vi "QPSK.vi"() -> ()   [LabVIEW 2018]
uses:
  <vilib>/addons/Modulation/Digital/General/MT Generate Bits (Galois, PN Order).vi
  <vilib>/addons/Modulation/Digital/Support/Common/Validators/mod_Generate Bits Validate.vi
  <vilib>/addons/Modulation/Analog/support/mod_Set Error Source.vi
  <vilib>/addons/Modulation/Digital/General/subVIs/mod_Generate Bits PN Sequence.vi
  <vilib>/addons/Modulation/niDMT.lvlib
panel:
  out "complex symbols":cdb[](array[numeric])
  in  "PN sequence order (9)":i32=9
  in  "total bits (128)":i32=128
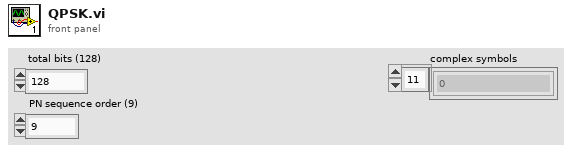
[diagram p1: front panel]
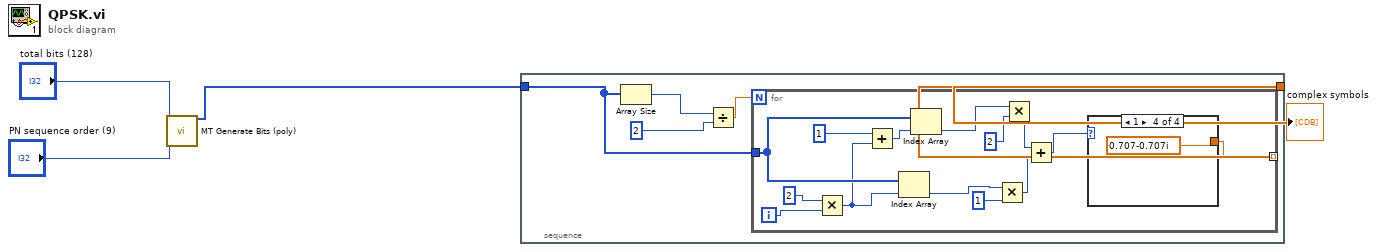
[diagram p0: block diagram]
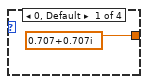
[diagram p2: hidden frame]
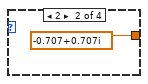
[diagram p3: hidden frame]
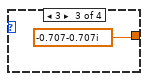
[diagram p4: hidden frame]
diagram:
  n1 = call-poly <vilib>:"MT Generate Bits (poly).vi"("total bits (128)"="total bits (128)", "PN sequence order (9)"="PN sequence order (9)") -> ("output bit stream"=w4:i8[])  [unwired: 11 in, 2 out]
  n2 = stacked-sequence {
    tunnel: [w5] -> w1
    tunnel: w4 -> [w9]
    frame #0 {
      n3 = Array Size(array=w9) -> (size(s)=w8:i32)
      n4 = Divide(x=w8, y=2) -> (x/y=w6:dbl)
      n5 = for {
        N: w6 -> [_]
        tunnel: w9 -> [w23]
        tunnel: [w11] -> w5 mode=indexing
        i -> [w18]
        n6 = Multiply(x=2, y=w18) -> (x*y=w20:i32)
        n7 = Add(x=1, y=w20) -> (x+y=w22:i32)
        n8 = Index Array(array=w23, index=w20) -> (element=w14:i8)
        n9 = Index Array(array=w23, index=w22) -> (element=w16:i8)
        n10 = Multiply(x=w14, y=1) -> (x*y=w12:i32)
        n11 = Multiply(x=w16, y=2) -> (x*y=w13:i32)
        n12 = Add(x=w13, y=w12) -> (x+y=w10:i32)
        n13 = case shown="1" w10 {
          tunnel: [cdb 0.707+0.707i cdb -0.707+0.707i cdb -0.707-0.707i cdb 0.707-0.707i] -> w11
          frame 0, Default {
          }
          frame 2 {
          }
          frame 3 {
          }
          frame 1 {
          }
        }
      }
    }
  }
  "complex symbols" <- w1
